vi "Load Sequence from file.vi"(8 "error in (no error)":errorcluster, 11 "Sequence file path\n(file dialog if empty)":path=path "D:/martin/QPsw - github/QuPMX/seqtest") -> (0 "error out":errorcluster, 1 "Timing\ndelay":u32[](array[numeric]) min=1 max=255 step=1, 3 "Sequence":bool[][](array[boolean]))   [LabVIEW 2020, in "QuPMXdriver.lvlib"]
doc: "Loads sequences represented as bytes from a simple tab delimited text file."
uses:
  QuPMXdriver.lvlib
  <vilib>/Utility/file.llb/Read Delimited Spreadsheet (I64).vi
panel:
  # "Slave index"
  # "1              2               3              4                5               6"
  # "Channel index"
  # "1     2       3      4       5      6      7       8      9     10     11    12"
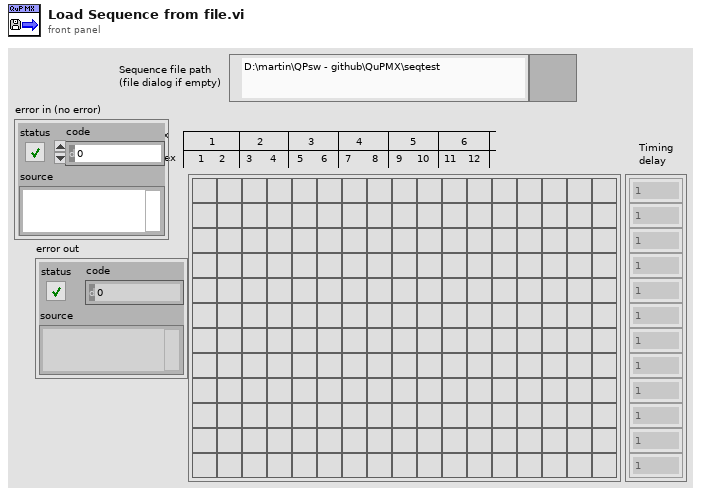
[diagram p1: front panel]
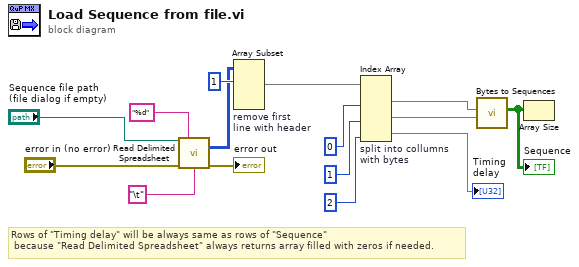
[diagram p0: block diagram]
diagram:
  # "Rows of \"Timing delay\" will be always same as rows of \"Sequence\"\n because \"Read Delimited Spreadsheet\" always returns array filled with zeros if needed."
  n1 = call-poly <vilib>:"Read Delimited Spreadsheet.vi"("file path (dialog if empty)"="Sequence file path\n(file dialog if empty)", "format (%d)"="%d", "error in (no error)"="error in (no error)", "delimiter (\\t)"="\t" ("delimiter (\\t)")) -> ("all rows"=w3:i64[][], "error out"=→"error out":errorcluster)  [unwired: 6 in, 4 out]
  n2 = Array Subset "remove first\nline with header"(array=w3, index (row)=1 ("index")) -> (w12:i64[][])  [unwired: 3 in]
  n3 = Index Array "split into collumns\nwith bytes"(array=w12, index (col) #1=0 ("disabled index (col)"), index (col) #2=1 ("disabled index (row)"), index (col) #3=2 ("index (row)")) -> (element #1=w7:i64[], element #2=w6:i64[], element #3=→"Timing\ndelay":i64[])  [unwired: 3 in]
  n4 = call "Bytes to Sequences.vi"("Ch. bytes 2"=w6, "Ch. bytes 1"=w7) -> ("Array"=w5:bool[][])  [unwired: 9 in]
  "Sequence" <- w5
  n5 = Array Size(array=w5) -> ()  [unwired: 1 out]
